vi "monthtoDateAll.vi"(9 "End Date":string="2014/11/13", 10 "From Date":string="2014/11/01") -> (1 "Table Control":string[][](table), 2 "output array":string[][](array[string]))   [LabVIEW 2012]
uses:
  <vilib>/addons/database/Auxilliary.llb/DB Tools Cursor Type.ctl
  <vilib>/addons/database/Connection.llb/DB Tools Open Connec (Path).vi
  <vilib>/addons/database/Connection.llb/Conn Execute.vi
  <vilib>/addons/database/Recordset.llb/Rec Fetch Recordset Data (R).vi
  <vilib>/addons/database/Recordset.llb/Rec Destroy - Connection.vi
  <vilib>/addons/database/_DB Variant To Data/Database Variant To Data.xnode
  <vilib>/addons/database/NI_Database_API.lvlib
panel:
  out "error out":errorcluster
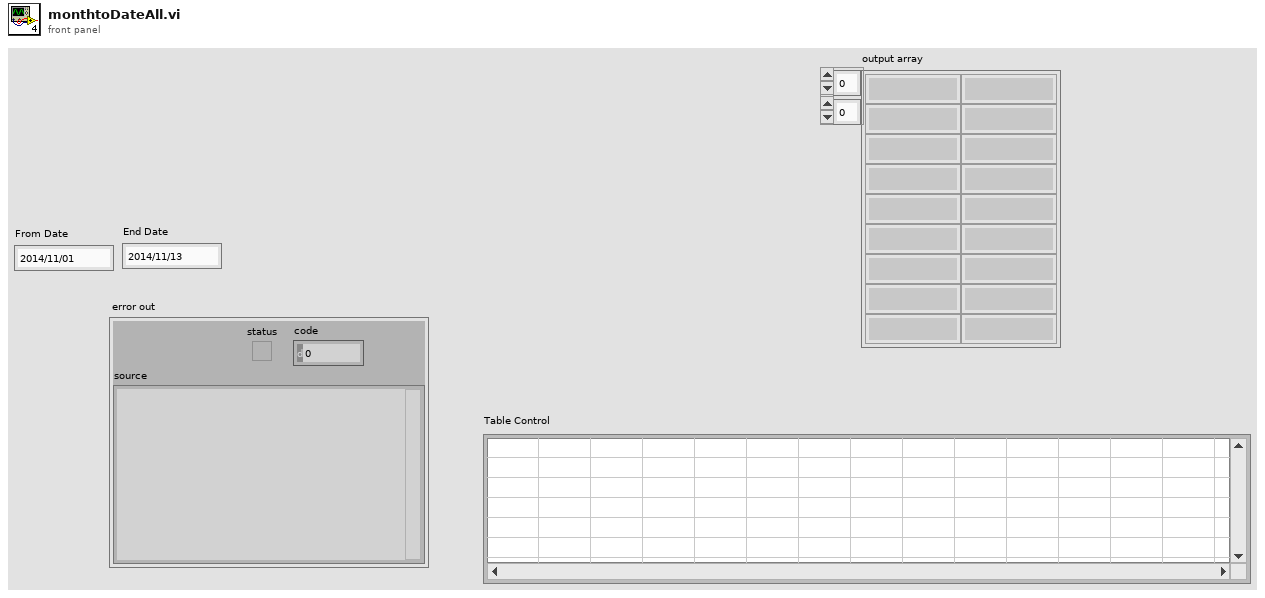
[diagram p1: front panel]
types:
  T1 = typedef "NI_Database_API.lvlib/DB Tools Cursor Type.ctl" = enum16{"forward-only", "keyset", "dynamic", "static"}
  T2 = typedef "NI_Database_API.lvlib/Conn ObjectReference.ctl" = refnum<k1>
  T3 = typedef "NI_Database_API.lvlib/Rec ObjectReference.ctl" = refnum<k1>
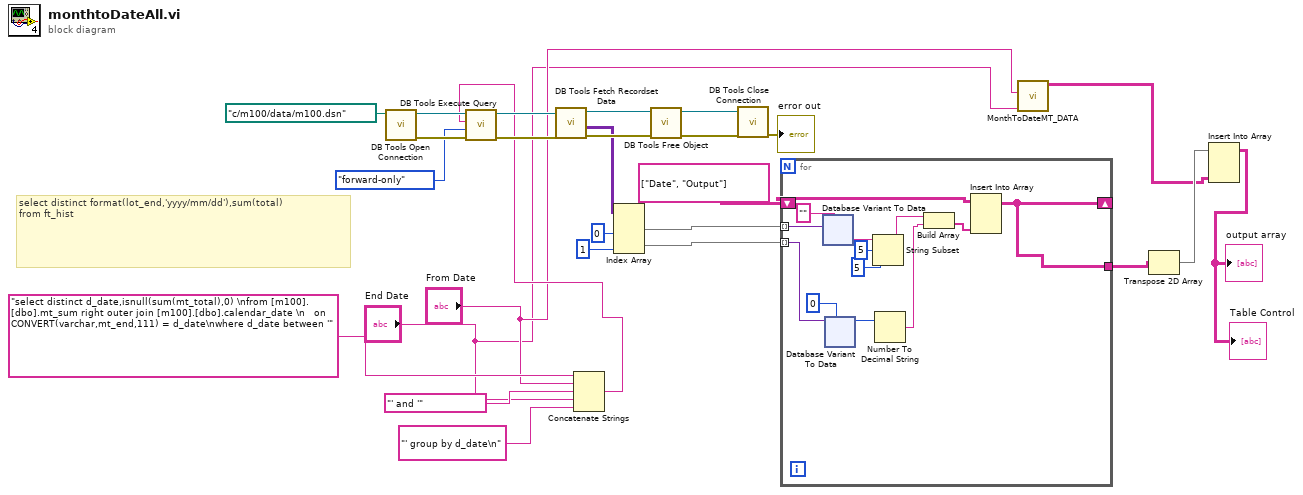
[diagram p0: block diagram]
diagram:
  # "select distinct format(lot_end,'yyyy/mm/dd'),sum(total)\nfrom ft_hist"
  n1 = call-poly <vilib>:"DB Tools Open Connection.vi"("connection information"=path "c:/m100/data/m100.dsn") -> ("error out"=w20:errorcluster, "connection reference"=w21:T2)  [unwired: 7 in]
  n2 = Concatenate Strings("select distinct d_date,isnull(sum(mt_total),0) \nfrom [m100].[dbo].mt_sum right outer join [m100].[dbo].calendar_date \n   on CONVERT(varchar,mt_end,111) = d_date\nwhere d_date between '" ("SQL query"), "From Date", "' and '" ("string"), "End Date", "' group by d_date\n" ("string")) -> (w8:string)
  n3 = call-poly <vilib>:"DB Tools Execute Query.vi"("error in (no error)"=w20, "cursor type"=DB_Tools_Cursor_Type."forward-only", "SQL query"=w8, "connection reference"=w21) -> ("error out"=w22:errorcluster, "recordset reference"=w23:T3)  [unwired: 4 in]
  n4 = call-poly <vilib>:"DB Tools Fetch Recordset Data.vi"("error in (no error)"=w22, "recordset reference"=w23) -> ("error out"=w24:errorcluster, "recordset data"=w13:variant[][], "recordset reference out"=w25:T3)  [unwired: 3 in]
  n5 = Index Array(array=w13, index (col) #1=0 ("disabled index (col)"), index (col) #2=1 ("index (col)")) -> (element #1=w16:variant[], element #2=w15:variant[])  [unwired: 2 in]
  n6 = call-poly <vilib>:"DB Tools Free Object.vi"("error in (no error)"=w24, "recordset reference"=w25) -> ("error out"=w27:errorcluster, "connection reference"=w26:T2)  [unwired: 8 in]
  n7 = call <vilib>:"DB Tools Close Connection.vi"("error in (no error)"=w27, "connection reference"=w26) -> ("error out"=→"error out":errorcluster)  [unwired: 5 in]
  n8 = for {
    tunnel: w16 -> [w40] mode=indexing
    tunnel: w15 -> [w39] mode=indexing
    shift-right: [w33] -> _
    shift-left: string[][] [["Date", "Output"]] ("array") -> [w34]
    tunnel: [w33] -> w7
    n9 = xnode "Database Variant To Data"("database variant"=w40, "type"="") -> ("data"=w32:string)  [unwired: 1 in, 1 out]
    n10 = xnode "Database Variant To Data"("database variant"=w39, "type"=0) -> ("data"=w28:i32)  [unwired: 1 in, 1 out]
    n11 = String Subset(string=w32, offset (0)=5, length (rest)=5 ("length (rest)")) -> (substring=w31:string)
    n12 = Number To Decimal String(number=w28) -> (decimal integer string=w36:string)  [unwired: 1 in]
    n13 = Build Array(w31, w36) -> (w35:string[])
    n14 = Insert Into Array(array=w34, new element=w35) -> (w33:string[][])  [unwired: 2 in]
  }
  n15 = call "MonthToDateMT_DATA.vi"("End Date"="End Date", "From Date"="From Date") -> ("subarray"=w3:string[][])  [unwired: 9 in]
  n16 = Transpose 2D Array(2D array=w7) -> (transposed array=w4:string[][])
  n17 = Insert Into Array(array=w4, new element=w3) -> (→"output array" →"Table Control":string[][])  [unwired: 2 in]
